vi "get_typeDescriptor.vi"(0 "HGF_DIMCommand":refnum<class "HGF_DIMCommand.lvclass">, 5 "error in (no error)":errorcluster) -> (14 "dup HGF_DIMCommand":refnum<class "HGF_DIMCommand.lvclass">, 16 "typeDescriptor":string, 19 "error out":errorcluster)   [LabVIEW 2012, in "HGF_DIM.lvlib" / "HGF_DIMCommand.lvclass"]
uses:
  HGF_DIMCommand.lvclass
  HGF_DIMCommand.lvclass/HGF_DIMCommand.ctl
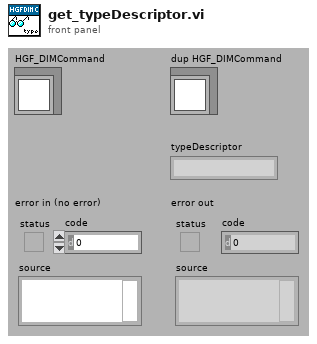
[diagram p1: front panel]
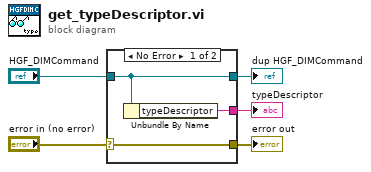
[diagram p0: block diagram]
diagram:
  n1 = case shown="No Error" "error in (no error)" {
    selector: "error in (no error)" -> [w8 w9]
    tunnel: [w8 w9] -> w4
    tunnel: [w7 w10] -> w2
    tunnel: "HGF_DIMCommand" -> [w7 w10]
    tunnel: [w6 _] -> w1
    frame No Error {
      n2 = Unbundle By Name(w7) -> ("typeDescriptor"=w6:string)
    }
    frame Error {
    }
  }
  "error out" <- w4
  "dup HGF_DIMCommand" <- w2
  "typeDescriptor" <- w1
